vi "ERD Read Test Generic (Boolean).vi"(0 "GEA2 Reference In":refnum<k24>, 5 "Standalone?":bool, 7 "ERD Number":u16=61699 format="%.0x", 9 "Expected T/F":enum16{"FALSE", "TRUE"}(ring), 11 "Error In":errorcluster) -> (4 "GEA2 Reference Out":refnum<k24>, 6 "Pass/Fail?":bool, 15 "Error Out":errorcluster)   [LabVIEW 2016, in "TLMB.lvlib"]
uses:
  Projects/TLMB.lvlib
  Q:/Common/DLLs/GEA3/GeaCommunication.dll
  Common/DLLs/GEA3/GeaCommunication.dll
  Common/LabVIEW GEA2 Toolkit/LabVIEW_GEA2_Toolkit.lvlibp/type defs/Source_Destination.ctl
  Common/LabVIEW GEA2 Toolkit/LabVIEW_GEA2_Toolkit.lvlibp/type defs/ERD Read Data In.ctl
  Common/LabVIEW GEA2 Toolkit/LabVIEW_GEA2_Toolkit.lvlibp/type defs/Data Type.ctl
  Common/LabVIEW GEA2 Toolkit/LabVIEW_GEA2_Toolkit.lvlibp
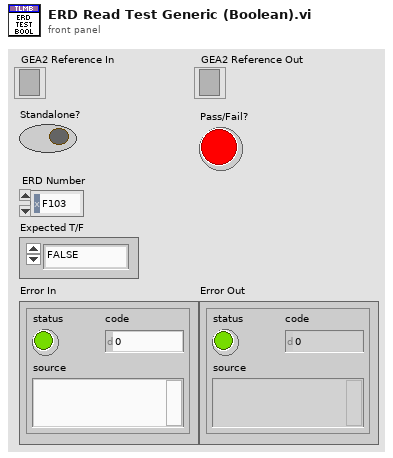
[diagram p1: front panel]
types:
  T1 = typedef "LabVIEW_GEA2_Toolkit.lvlibp/ERD Read Data In.ctl" = cluster{"ERD Number":u16, "Data Type":T2}
  T2 = typedef "LabVIEW_GEA2_Toolkit.lvlibp/Data Type.ctl" = enum16{"string", "boolean", "uint8_t", "uint16_t", "uint32_t", "uint64_t", "int8_t", "int16_t", "int32_t", "int64_t"}
  T3 = enum16{"string", "boolean", "uint8_t", "uint16_t", "uint32_t"}
  T4 = typedef "LabVIEW_GEA2_Toolkit.lvlibp/Source_Destination.ctl" = cluster{"Source":u8, "Destination":u8}
  T5 = typedef "LabVIEW_GEA2_Toolkit.lvlibp/ERD Read Data Out.ctl" = cluster{"ERD Number":u16, "Data":string}
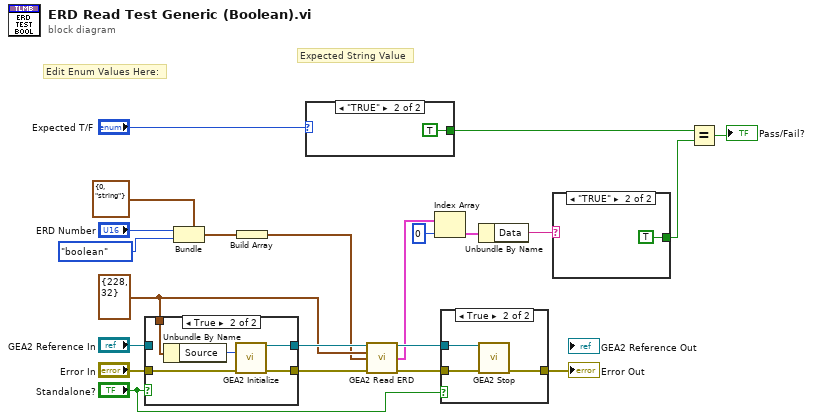
[diagram p0: block diagram]
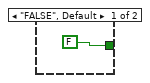
[diagram p2: hidden frame]
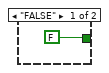
[diagram p3: hidden frame]
diagram:
  w14 = T4 {"Source"=228, "Destination"=32} ("GEA Inputs")
  # "Expected String Value"
  # "Edit Enum Values Here:"
  n1 = case shown="True" "Standalone?" {
    tunnel: "Error In" -> [w23 w29]
    tunnel: [w23 w28] -> w18
    tunnel: "GEA2 Reference In" -> [w24 _]
    tunnel: [w24 w27] -> w16
    tunnel: w14 -> [_ w25]
    frame False {
    }
    frame True {
      n2 = Unbundle By Name(w25) -> ("Source"=w26:u8)
      n3 = call "GEA2 Initialize.vi"("Source Address"=w26, "error in"=w29) -> ("GEA2 Reference Out"=w27:refnum<k24>, "error out"=w28:errorcluster)  [unwired: 11 in, 1 out]
    }
  }
  n4 = Bundle(cluster=T1 {"ERD Number"=0, "Data Type"=enum."string"} ("ERD Read Data In"), "ERD Number"="ERD Number", "Data Type"=T3."boolean") -> (w2:T1)
  n5 = Build Array(w2) -> (w1:T1[])
  n6 = case shown="\"TRUE\"" "Expected T/F" {
    tunnel: [FALSE TRUE] -> w9
    frame "FALSE" {
    }
    frame "TRUE" {
    }
  }
  n7 = call "GEA2 Read ERD.vi"("GEA2 Reference In"=w16, "GEA Inputs"=w14, "Read ERD List"=w1, "Error In"=w18) -> ("GEA2 Reference Out"=w15:refnum<k24>, "ERD Data Out"=w13:T5[], "Error Out"=w17:errorcluster)  [unwired: 8 in, 1 out]
  n8 = Index Array(array=w13, index=0) -> (element=w11:T5)
  n9 = case shown="True" "Standalone?" {
    tunnel: [w32 w35] -> w20
    tunnel: w17 -> [w32 w34]
    tunnel: w15 -> [_ w33]
    frame False {
    }
    frame True {
      n10 = call "GEA2 Stop.vi"("GEA2 Reference In"=w33, "Error In"=w34) -> ("Error Out"=w35:errorcluster)  [unwired: 13 in]
    }
  }
  "Error Out" <- w20
  n11 = Unbundle By Name(w11) -> ("Data"=w7:string)
  n12 = case shown="\"TRUE\"" w7 {
    tunnel: [FALSE TRUE] -> w6
    frame "FALSE", Default {
    }
    frame "TRUE" {
    }
  }
  n13 = Equal?(x=w9, y=w6) -> (x = y?=→"Pass/Fail?":bool)
